vi "niFpgaPeriodTemplate.vi"(0 "input data":fxp<+/-,16,16>, 1 "reset":bool, 5 "threshold level":fxp<+/-,16,16>, 7 "hysteresis":fxp<+/-,16,16>, 9 "direction":u8(ring) items=["falling", "rising"]) -> (4 "period (samples)":fxp<+,32,16>, 6 "timeout":bool, 8 "crossing":bool, 10 "output valid":bool)   [LabVIEW 2017]
uses:
  <vilib>/Platform/TimedLoop/XDataNode/timing_clust.ctl
  <vilib>/Platform/TimedLoop/XDataNode/nitl_modes.ctl
  <vilib>/Platform/TimedLoop/XDataNode/wakeup.ctl
  <vilib>/Platform/TimedLoop/XDataNode/XDataNode.xnode
  <vilib>/Platform/TimedLoop/XDataNode/XDNodeRunTimeDep.lvlib
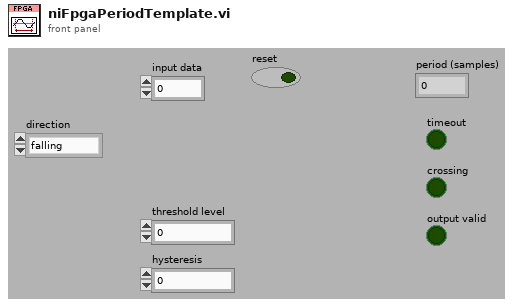
[diagram p1: front panel]
types:
  T1 = typedef "XDNodeRunTimeDep.lvlib/timing_clust.ctl" = cluster{"Expected End [f-1]":u64, "Actual End [f-1]":u64, "Finished Late? [f-1]":bool, "Expected End [i-1]":u64, "Actual End [i-1]":u64, "Finished Late? [i-1]":bool, "Expected Start [i]":u64, "Actual Start [i]":u64, "Expected Start [f]":u64, "Actual Start [f]":u64, "Source Name":string, "Structure Name":string, "Period":i64, "Deadline":i64, "Offset":i64, "Start":i64, "Priority":i32, "Timeout":i32, "Mode":T2, "Wakeup Reason":T3, "Error":errorcluster, "Source Type":string, "Secondary Source Type":string, "Global End Time":u64, "Global Start Time":u64, "Frame Duration":u64, "Iteration Duration":u64, "Assigned CPU":i32, "I/O Scan Engine Mode":u32}
  T2 = typedef "XDNodeRunTimeDep.lvlib/nitl_modes.ctl" = enum32{"No Change", "Process missed periods, maintain original phase", "Discard missed periods, maintain original phase", "Process missed periods, ignore original phase", "Discard missed periods, ignore original phase"}
  T3 = typedef "XDNodeRunTimeDep.lvlib/wakeup.ctl" = enum32{"Normal", "Aborted", "Asynchronous wakeup", "Timing source error", "Timed loop error", "Timeout"}
  T4 = typedef "niFPGA Threshold Crossing State.ctl" = cluster{"level":bool[], "rising?":bool, "hi hyst met?":bool, "lo hyst met?":bool, "gt threshold":bool, "lt threshold":bool}
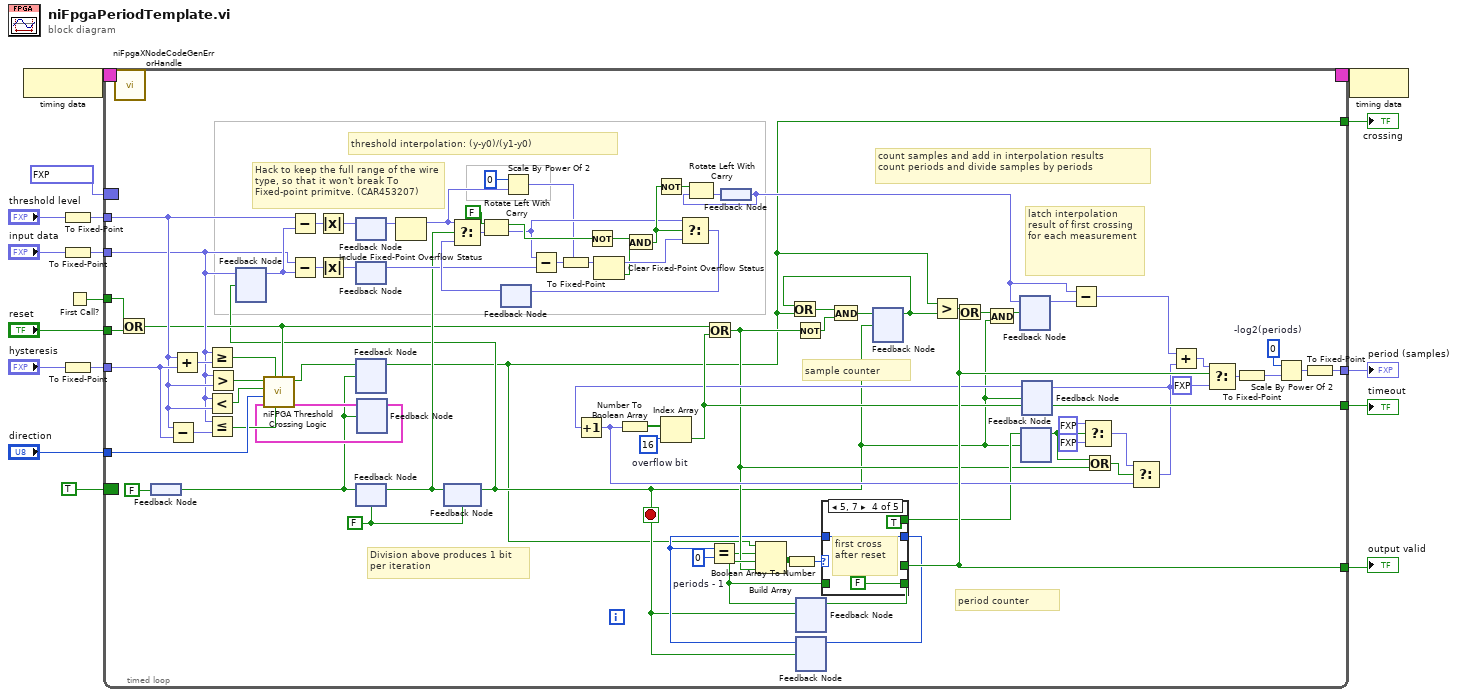
[diagram p0: block diagram]
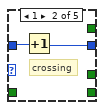
[diagram p3: hidden frame]
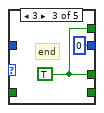
[diagram p4: hidden frame]
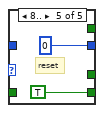
[diagram p5: hidden frame]
diagram:
  n1 = node-c288() -> (w16:T1)
  n2 = To Fixed-Point(number="threshold level") -> (fixed-point=w4:fxp<+/-,16,16>)  [unwired: 1 in]
  n3 = To Fixed-Point(number="input data") -> (fixed-point=w3:fxp<+/-,16,16>)  [unwired: 1 in]
  n4 = To Fixed-Point(number="hysteresis") -> (fixed-point=w2:fxp<+/-,16,16>)  [unwired: 1 in]
  n5 = First Call?() -> (First Call?: T/F=w1:bool)
  n6 = timed-loop "SCTL" {
    tunnel: [w87] -> w7
    tunnel: [w102] -> w17
    timing: w16 -> [_]
    timing-out: [_] -> w15
    tunnel: [w101] -> w14
    tunnel: w3 -> [w73]
    tunnel: "direction" -> [w93]
    tunnel: w4 -> [w74]
    tunnel: w2 -> [w100]
    tunnel: "reset" -> [w99]
    border: TRUE -> [_]
    tunnel: [w21] -> w6
    border: fxp<+,8,0> 0.0 -> [_]
    tunnel: w1 -> [w60]
    stop <- w23 stop-if-true
    w22 = FALSE
    w39 = i16 0  # -log2(periods)
    w41 = u16 0  # periods - 1
    w51 = 16  # overflow bit
    # "Hack to keep the full range of the wire type, so that it won't break To Fixed-point primitve. (CAR453207)"
    # "period counter"
    # "sample counter"
    # "count samples and add in interpolation results\ncount periods and divide samples by periods"
    # "latch interpolation result of first crossing for each measurement"
    # "Division above produces 1 bit \nper iteration"
    # "threshold interpolation: (y-y0)/(y1-y0)"
    n7 = Or(x=w60, y=w99) -> (x .or. y?=w59:bool)
    n8 = feedback-in #1(FALSE) -> ()
    n9 = feedback #1() -> (w64:bool)
    n10 = Subtract(x=w74, y=w100) -> (x-y=w98:fxp<+/-,17,17>)
    n11 = Add(x=w74, y=w100) -> (x+y=w97:fxp<+/-,17,17>)
    n12 = Greater Or Equal?(x=w73, y=w97) -> (x >= y?=w96:bool)
    n13 = Less?(x=w73, y=w74) -> (x < y?=w94:bool)
    n14 = Less Or Equal?(x=w73, y=w98) -> (x <= y?=w92:bool)
    n15 = Greater?(x=w73, y=w74) -> (0:w95:bool)
    n16 = feedback #2() -> (w84:fxp<+/-,16,16>)  [unwired: 1 in]
    n17 = Subtract(x=w74, y=w84) -> (x-y=w85:fxp<+/-,17,17>)
    n18 = Subtract(x=w73, y=w84) -> (x-y=w86:fxp<+/-,17,17>)
    n19 = Absolute Value(x=w85) -> (abs(x)=w67:fxp<+,16,16>)
    n20 = Absolute Value(x=w86) -> (abs(x)=w68:fxp<+,16,16>)
    n21 = feedback-in #3(w67) -> ()
    n22 = feedback #3() -> (w66:fxp<+,16,16>)  [unwired: 1 in]
    n23 = feedback-in #4(w68) -> ()
    n24 = feedback #4() -> (w65:fxp<+,16,16>)  [unwired: 1 in]
    n25 = feedback #5() -> (w21:bool)  [unwired: 1 in]
    n26 = feedback-in #6(w64) -> ()
    n27 = feedback #6(w22) -> (w63:bool)
    n28 = feedback #7() -> (w90:T4)  [unwired: 1 in]
    n29 = call <vilib>:"niFPGA Threshold Crossing Logic.vi"("reset"=w59, "le low ref"=w92, "ge high ref"=w96, "state in"=w90, "direction"=w93, "lt threshold"=w94, "gt threshold"=w95) -> ("state out"=w91:T4, "crossing"=w89:bool)  [unwired: 3 in]
    n30 = feedback-in #5(w89, w64) -> ()
    n31 = feedback-in #7(w91, w64) -> ()
    n32 = Include Fixed-Point Overflow Status(3:w66) -> (1:w20:fxp<+,16,16>)  [unwired: 1 in]
    n33 = feedback-in #8(w63) -> ()
    n34 = feedback #8(w22) -> (w23:bool)
    n35 = feedback-in #2(w73, w23) -> ()
    n36 = feedback #9() -> (w69:fxp<+,16,16>)  [unwired: 1 in]
    n37 = Select(t=w20, s=w63, f=w69) -> (s? t:f=w71:fxp<+,16,16>)
    n38 = Rotate Left With Carry(2:w71, 3:FALSE ("carry")) -> (0:w70:fxp<+,16,16>, 1:w81:bool)
    n39 = Scale By Power Of 2(n=i16 0, x=w20) -> (x*2^n=w18:fxp<+,16,16>)
    n40 = Subtract(x=w70, y=w65) -> (x-y=w78:fxp<+/-,17,17>)
    n41 = To Fixed-Point(fixed-point type=w18, number=w78) -> (fixed-point=w72:fxp<+,16,16>)
    n42 = Not(x=w81) -> (.not. x?=w80:bool)
    n43 = Clear Fixed-Point Overflow Status(3:w72) -> (0:w76:bool, 1:w77:fxp<+,16,16>)
    n44 = And(x=w80, y=w76) -> (x .and. y?=w79:bool)
    n45 = Not(x=w79) -> (.not. x?=w83:bool)
    n46 = Select(t=w70, s=w79, f=w77) -> (s? t:f=w75:fxp<+,16,16>)
    n47 = feedback-in #9(w75) -> ()
    n48 = feedback #10() -> (w61:fxp<+,8,0>)
    n49 = Rotate Left With Carry(2:w61, 3:w83) -> (0:w62:fxp<+,8,0>)  [unwired: 1 out]
    n50 = feedback-in #10(w62) -> ()
    n51 = feedback #11() -> (w54:bool)  [unwired: 1 in]
    n52 = feedback #12() -> (w42:u16)  [unwired: 1 in]
    n53 = Equal?(x=w42, y=w41) -> (x = y?=w43:bool)
    n54 = feedback #13() -> (w32:bool)  [unwired: 1 in]
    n55 = Or(x=w32, y=w21) -> (x .or. y?=w35:bool)
    n56 = Greater?(x=w21, y=w32) -> (0:w37:bool)
    n57 = feedback #14() -> (w31:fxp<+,8,0>)  [unwired: 1 in]
    n58 = feedback #15() -> (w38:bool)  [unwired: 1 in]
    n59 = feedback #16() -> (w47:fxp<+,25,25>)  [unwired: 1 in]
    n60 = Increment(x=w47) -> (x+1=w53:fxp<+,25,25>)
    n61 = Number To Boolean Array(number=w53) -> (Boolean array=w52:bool[])
    n62 = Index Array(array=w52, index=w51) -> (element=w101:bool)
    n63 = Or(x=w59, y=w101) -> (x .or. y?=w45:bool)
    n64 = Build Array(w21, w43, w54, w45) -> (w58:bool[])
    n65 = Boolean Array To Number(Boolean array=w58) -> (number=w57:u8)
    n66 = Not(x=w45) -> (.not. x?=w36:bool)
    n67 = case shown="5, 7" w57 {
      tunnel: [w103 _ _ FALSE TRUE] -> w56
      tunnel: w42 -> [w104 w106 _ w111 _]
      tunnel: [w104 w105 u16 0 w111 u16 0] -> w55
      tunnel: w54 -> [w103 _ _ _ _]
      tunnel: [_ _ w107 _ _] -> w102
      tunnel: [_ _ w107 TRUE _] -> w46
      frame Default {
        # "wait for crossing"
      }
      frame 1 {
        # "crossing"
        n68 = Increment(x=w106) -> (x+1=w105:u16)
      }
      frame 3 {
        w107 = TRUE
        # "end"
      }
      frame 5, 7 {
        # "first cross after reset"
      }
      frame 8.. {
        # "reset"
      }
    }
    n69 = feedback-in #11(w56, w23) -> ()
    n70 = feedback-in #12(w55, w23) -> ()
    n71 = And(x=w35, y=w36) -> (x .and. y?=w33:bool)
    n72 = feedback-in #13(w33, w23) -> ()
    n73 = Or(x=w37, y=w102) -> (x .or. y?=w25:bool)
    n74 = And(x=w25, y=w23) -> (x .and. y?=w24:bool)
    n75 = feedback-in #14(w61, w24) -> ()
    n76 = feedback-in #15(w46, w23) -> ()
    n77 = Subtract(x=w61, y=w31) -> (x-y=w34:fxp<+/-,9,1>)
    n78 = Select(t=fxp<+,25,25> 1.0, s=w38, f=fxp<+,25,25> 0.0 ("t")) -> (s? t:f=w48:fxp<+,25,25>)
    n79 = Or(x=w38, y=w45) -> (x .or. y?=w44:bool)
    n80 = Select(t=w48, s=w44, f=w53) -> (s? t:f=w30:fxp<+,25,25>)
    n81 = feedback-in #16(w30, w23) -> ()
    n82 = Add(x=w34, y=w30) -> (x+y=w29:fxp<+/-,34,26>)
    n83 = Select(t=w29, s=w102, f=fxp<+/-,34,26> 0.0) -> (s? t:f=w40:fxp<+/-,34,26>)
    n84 = To Fixed-Point(number=w40) -> (fixed-point=w26:fxp<+/-,42,26>)  [unwired: 1 in]
    n85 = Scale By Power Of 2(n=w39, x=w26) -> (x*2^n=w27:fxp<+/-,42,26>)
    n86 = To Fixed-Point(number=w27) -> (fixed-point=w87:fxp<+,32,16>)  [unwired: 1 in]
  }
  "output valid" <- w17
  "period (samples)" <- w7
  "timeout" <- w14
  "crossing" <- w6
  n87 = call <vilib>:"niFpgaXNodeCodeGenErrorHandle.vi"() -> ()  [unwired: 1 in]
  n88 = node-c288(w15) -> ()
